vi "Toggle.vi"(8 "direction":enum16{"either", "false-true", "true-false"}(ring), 11 "Input":bool) -> (3 "Output":bool)   [LabVIEW 2016]
uses:
  <vilib>/ptbypt/NI_PtbyPt.lvlib
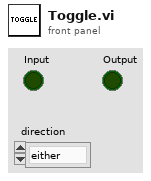
[diagram p1: front panel]
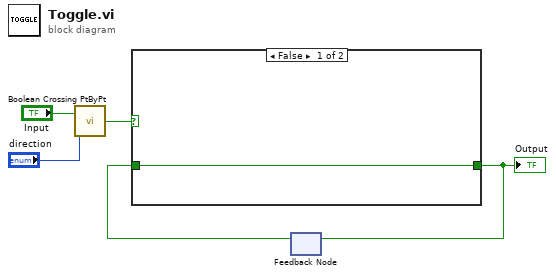
[diagram p0: block diagram]
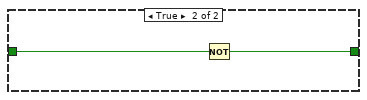
[diagram p2: hidden frame]
diagram:
  n1 = call <vilib>:"Boolean Crossing PtByPt.vi"("direction"="direction", "input"="Input") -> ("crossing"=w5:bool)  [unwired: 1 in]
  n2 = feedback #1() -> (w2:bool)  [unwired: 1 in]
  n3 = case shown="False" w5 {
    tunnel: [w6 w7] -> w1
    tunnel: w2 -> [w6 w8]
    frame False {
    }
    frame True {
      n4 = Not(x=w8) -> (.not. x?=w7:bool)
    }
  }
  "Output" <- w1
  n5 = feedback-in #1(w1) -> ()
